vi "HealthCheckIMU (1).vi"(9 "Numeric 3":dbl, 10 "Numeric 2":dbl, 11 "Numeric":dbl) -> (1 "Boolean 3":bool, 2 "Boolean 2":bool, 3 "Boolean":bool)   [LabVIEW 2017]
uses:
  NominalRangeGLOBAL.vi
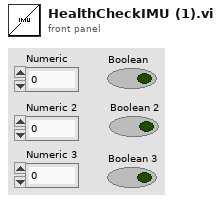
[diagram p1: front panel]
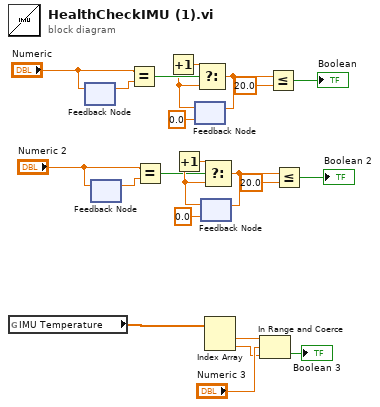
[diagram p0: block diagram]
diagram:
  n1 = global read "NominalRangeGLOBAL.vi" "IMU Temperature"() -> (w21:dbl[])
  n2 = feedback-in #1("Numeric") -> ()
  n3 = feedback #1() -> (w17:dbl)  [unwired: 1 in]
  n4 = feedback #2() -> (w2:dbl)  [unwired: 1 in]
  n5 = feedback-in #2("Numeric 2") -> ()
  n6 = Equal?(x="Numeric", y=w17) -> (x = y?=w16:bool)
  n7 = Equal?(x="Numeric 2", y=w2) -> (x = y?=w3:bool)
  n8 = feedback #3(0.0) -> (w14:dbl)
  n9 = Increment(x=w14) -> (x+1=w15:dbl)
  n10 = Select(t=w15, s=w16, f=w14) -> (s? t:f=w12:dbl)
  n11 = feedback-in #3(w12) -> ()
  n12 = feedback #4(0.0) -> (w5:dbl)
  n13 = Increment(x=w5) -> (x+1=w4:dbl)
  n14 = Select(t=w4, s=w3, f=w5) -> (s? t:f=w7:dbl)
  n15 = feedback-in #4(w7) -> ()
  n16 = Index Array(array=w21) -> (element #1=w20:dbl, element #2=w19:dbl)  [unwired: 2 in]
  n17 = In Range and Coerce(upper limit=w20, x="Numeric 3", lower limit=w19) -> (In Range?=→"Boolean 3":bool)  [unwired: 1 out]
  n18 = Less Or Equal?(x=w12, y=20.0) -> (x <= y?=→"Boolean":bool)
  n19 = Less Or Equal?(x=w7, y=20.0) -> (x <= y?=→"Boolean 2":bool)
